vi "Extract_ROIs_in Clusterform.vi"(9 "Norm. XYZ Coordinates":T1[](array[typedef]) {"Apparent Frame Size" format="%#_6f"; "Original FOV (um)" format="%#_6f"; "Pixels per miniscan" format="%#_6f"; "Dwell Time per pixel" format="%#_6f"; "Resolution" format="%#_6f"; "ROI group ID" format="%#_6f"; "Laser Power (%)" format="%#_6f"; "Zoom" format="%#_6f"; "Frame Size" format="%#_6f"; "Number of lines" format="%#_6f"; "Composite ID" format="%#_6f"; "Angle (deg)" format="%#_6f"; "ROI Time (ns)" format="%#_6f"; "ROI ID" format="%#_6f"; "Pixels in ROI" format="%#_6f"; "ROI index" format="%#_6f"; "Z stop" format="%#_6f"; "Y stop" format="%#_6f"; "X stop" format="%#_6f"; "Z start" format="%#_6f"; "X start" format="%#_6f"; "Y start" format="%#_6f"}) -> (0 "miniScan_Indices":dbl[](array[numeric]), 1 "miniScan_Coordinates":T2, 2 "POI_Indices":dbl[](array[numeric]), 3 "Point_Coordinates":T2)   [LabVIEW 2020]
uses:
  Typedefs/ROI XY coordinates cluster.ctl
  Visualisation/Functional Imaging Viewer/Typedefs/ROI parameters data type.ctl
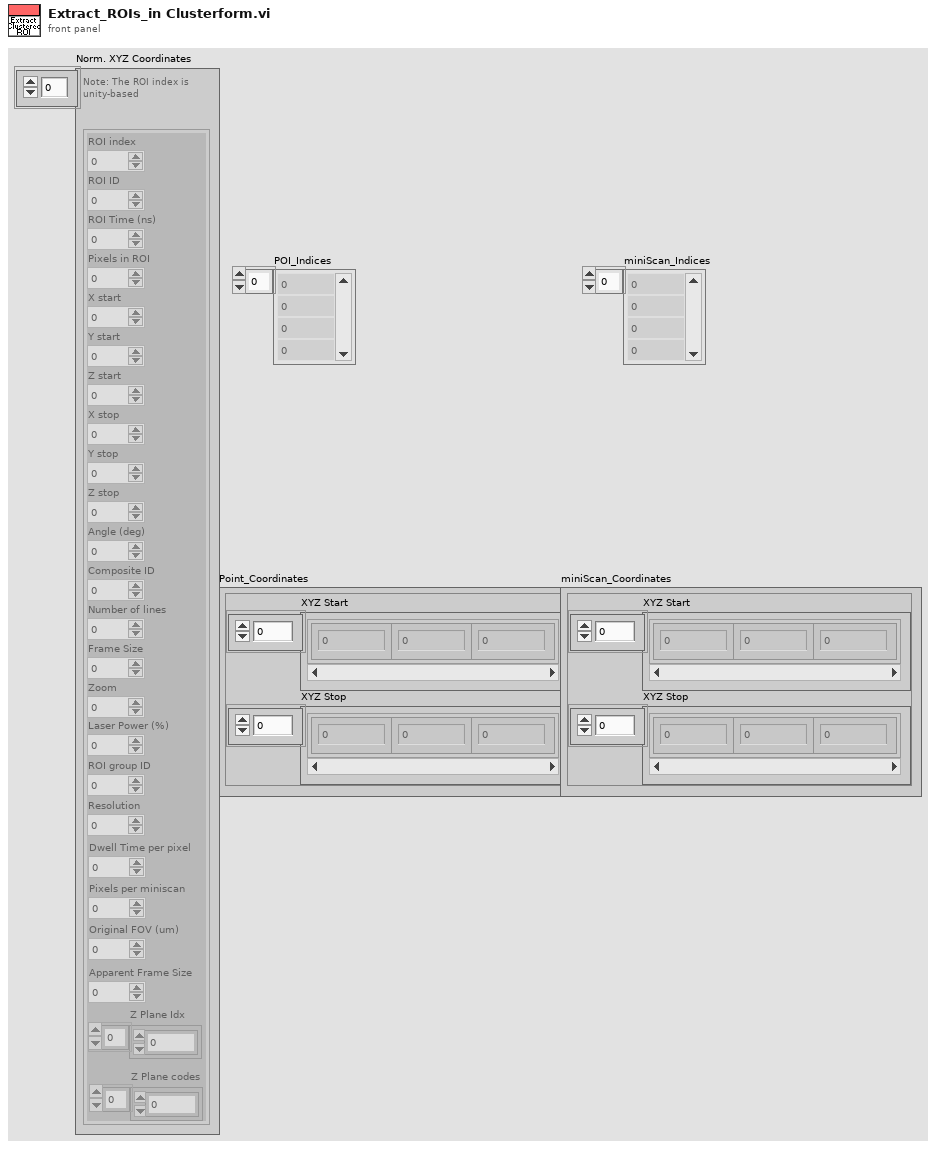
[diagram p1: front panel]
types:
  T1 = typedef "ROI parameters data type.ctl" = cluster{"ROI index":dbl, "ROI ID":dbl, "ROI Time (ns)":dbl, "Pixels in ROI":dbl, "X start":dbl, "Y start":dbl, "Z start":dbl, "X stop":dbl, "Y stop":dbl, "Z stop":dbl, "Angle (deg)":dbl, "Composite ID":dbl, "Number of lines":dbl, "Frame Size":dbl, "Zoom":dbl, "Laser Power (%)":dbl, "ROI group ID":dbl, "Resolution":dbl, "Dwell Time per pixel":dbl, "Pixels per miniscan":dbl, "Original FOV (um)":dbl, "Apparent Frame Size":dbl, "Z Plane Idx":i32[], "Z Plane codes":i32[]}
  T2 = typedef "ROI XY coordinates cluster.ctl" = cluster{"XYZ Start":cluster{"X":sgl, "Y":sgl, "Z":sgl}[], "XYZ Stop":cluster{"X":sgl, "Y":sgl, "Z":sgl}[]}
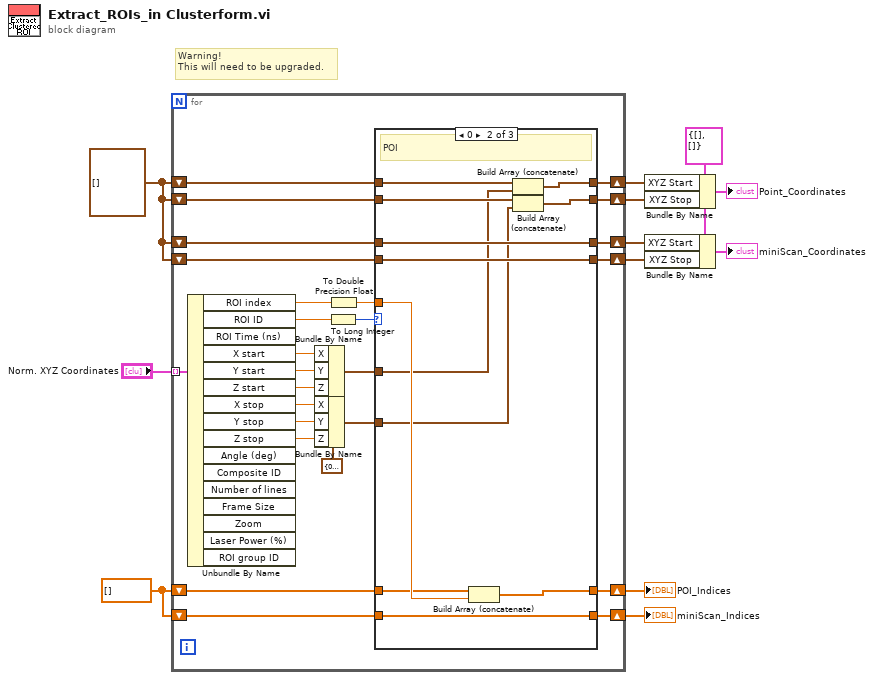
[diagram p0: block diagram]
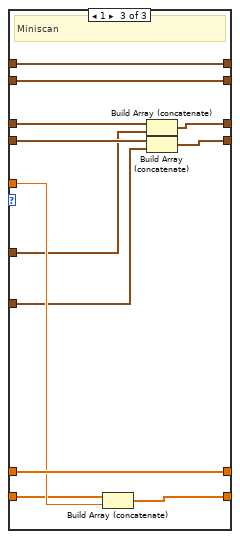
[diagram p3: hidden frame]
diagram:
  w1 = T2 {"XYZ Start"=[], "XYZ Stop"=[]} ("ROI Coordinates")
  w11 = cluster{"X":dbl, "Y":dbl, "Z":dbl}[] [] ("XYZ Coordinates")
  w12 = dbl[] []
  # "Warning!\nThis will need to be upgraded."
  n1 = for {
    tunnel: "Norm. XYZ Coordinates" -> [w38] mode=indexing
    shift-right: [w35] -> w10
    shift-left: w12 -> [w34]
    shift-right: [w33] -> w9
    shift-left: w12 -> [w32]
    shift-right: [w24] -> w8
    shift-left: w11 -> [w31]
    shift-right: [w30] -> w6
    shift-left: w11 -> [w29]
    shift-right: [w28] -> w7
    shift-left: w11 -> [w27]
    shift-right: [w26] -> w5
    shift-left: w11 -> [w25]
    w22 = cluster{"X":dbl, "Y":dbl, "Z":dbl} {"X"=0.0, "Y"=0.0, "Z"=0.0} ("XYZ")
    n2 = Unbundle By Name(w38) -> ("ROI index"=w36:dbl, "ROI ID"=w37:dbl, "X start"=w21:dbl, "Y start"=w20:dbl, "Z start"=w19:dbl, "X stop"=w18:dbl, "Y stop"=w17:dbl, "Z stop"=w16:dbl)  [unwired: 8 out]
    n3 = Bundle By Name(cluster=w22, "X"=w21, "Y"=w20, "Z"=w19) -> (w15:cluster{"X":dbl, "Y":dbl, "Z":dbl})
    n4 = Bundle By Name(cluster=w22, "X"=w18, "Y"=w17, "Z"=w16) -> (w14:cluster{"X":dbl, "Y":dbl, "Z":dbl})
    n5 = To Long Integer(number=w37) -> (32bit integer=w13:i32)
    n6 = To Double Precision Float(number=w36) -> (double precision float=w23:dbl)
    n7 = case shown="0" w13 {
      tunnel: w23 -> [_ w56 w67]
      tunnel: [w40 w55 w68] -> w35
      tunnel: w34 -> [w40 w54 w68]
      tunnel: [w39 w53 w66] -> w33
      tunnel: w32 -> [w39 w53 w65]
      tunnel: w31 -> [w44 w51 w64]
      tunnel: [w42 w50 w63] -> w30
      tunnel: w29 -> [w42 w50 w62]
      tunnel: [w43 w49 w61] -> w28
      tunnel: w27 -> [w43 w48 w61]
      tunnel: [w41 w47 w60] -> w26
      tunnel: w25 -> [w41 w47 w59]
      tunnel: [w44 w52 w64] -> w24
      tunnel: w15 -> [_ w46 w58]
      tunnel: w14 -> [_ w45 w57]
      frame Default {
      }
      frame 0 {
        # "POI"
        n8 = Build Array (concatenate)(w54, w56) -> (w55:dbl[])
        n9 = Build Array (concatenate)(w51, w46) -> (w52:cluster{"X":dbl, "Y":dbl, "Z":dbl}[])
        n10 = Build Array (concatenate)(w48, w45) -> (w49:cluster{"X":dbl, "Y":dbl, "Z":dbl}[])
      }
      frame 1 {
        # "Miniscan"
        n11 = Build Array (concatenate)(w65, w67) -> (w66:dbl[])
        n12 = Build Array (concatenate)(w62, w58) -> (w63:cluster{"X":dbl, "Y":dbl, "Z":dbl}[])
        n13 = Build Array (concatenate)(w59, w57) -> (w60:cluster{"X":dbl, "Y":dbl, "Z":dbl}[])
      }
    }
  }
  "POI_Indices" <- w10
  "miniScan_Indices" <- w9
  n14 = Bundle By Name(cluster=w1, "XYZ Start"=w8, "XYZ Stop"=w7) -> (→"Point_Coordinates":T2)
  n15 = Bundle By Name(cluster=w1, "XYZ Start"=w6, "XYZ Stop"=w5) -> (→"miniScan_Coordinates":T2)
